vi "IMIC_SetZMoving.vi"(0 "X-speed":dbl, 5 "handle":u64) -> (1 "handle out":u64, 2 "output param":T1(ring))   [LabVIEW 2011]
uses:
  tillimic64.dll
panel:
  # "never used"
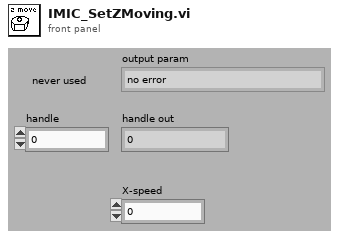
[diagram p1: front panel]
types:
  T1 = enum16{"no error", "missing axis", "missing Z axis", "missing Filter", "iMic not initialized", "no property", "wrong handle", "protocol not finished", "user parameter to long (>32 bits)", "no user parameter handle", "failed to open comport", "failed to initialize"}
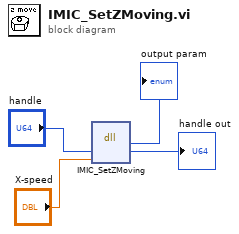
[diagram p0: block diagram]
diagram:
  n1 = dll-call lib="C:/Program Files/colibri/Drivers/TILLPhotonics/tillimic*.*" fn="IMIC_SetZMoving"("handle"="handle", "speed"="X-speed") -> ("return type"=→"output param":i32, "handle"=→"handle out":u64)  [unwired: 4 in, 2 out]
